vi "Basic Example.vi"() -> ()   [LabVIEW 2017]
uses:
  Promise/Promise/Promise.lvclass/Promise.ctl
  2bec5435-86af-4869-92e2-362b84164951.vi
  9c3bbcd6-5453-4f9a-927e-3563458ec675.vi
  08d1302d-8b04-4b09-9bc2-546fd279247c.vi
  Promise/Promise/Resolve Promise.vi
  <vilib>/Utility/error.llb/Error Cluster From Error Code.vi
  Promise/Promise/Wait on Promise.vi
  Promise/Promise/Promise.lvclass
panel:
  in  "Set Button":bool
  in  "String":string
  out "Value 2":string
  out "Value":string
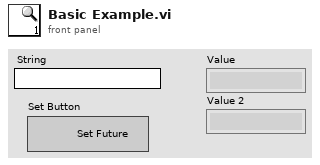
[diagram p1: front panel]
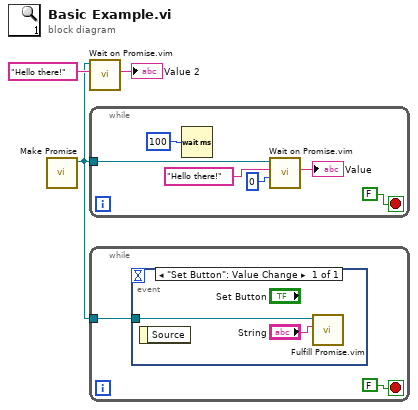
[diagram p0: block diagram]
diagram:
  n1 = call "Make Promise.vi"() -> ("Promise out"=w1:refnum<class "Promise.lvclass">)  [unwired: 9 in, 2 out]
  n2 = call "Wait on Promise.vim"("Default Value"="Hello there!", "Promise in"=w1) -> ("Value"=→"Value 2":string)  [unwired: 6 in, 3 out]
  n3 = while {
    tunnel: w1 -> [w4]
    stop <- FALSE stop-if-true
    n4 = Wait (ms)(milliseconds to wait=u32 100) -> ()  [unwired: 1 out]
    n5 = call "Wait on Promise.vim"("timeout in ms (-1)"=0, "Default Value"="Hello there!", "Promise in"=w4) -> ("Value"=→"Value":string)  [unwired: 5 in, 3 out]
  }
  n6 = while {
    tunnel: w1 -> [w10]
    stop <- FALSE stop-if-true
    n7 = event shown="[0] \"Set Button\": Value Change" {
      selector: _ -> [_]
      dyn-events: _ -> [_]
      timeout: _ -> [_]
      tunnel: w10 -> [w12]
      event "Set Button": Value Change {
        n8 = event-data() -> ()  [unwired: 1 in, 1 out]
        n9 = call "Fulfill Promise.vim"("Value"="String", "Promise in"=w12) -> ()  [unwired: 8 in, 2 out]
      }
    }
  }
